vi "Get COM List.vi"(8 "error in (no error)":errorcluster) -> (0 "error out":errorcluster, 1 "raw string list":string, 2 "COM ports count":i32, 3 "COM list":T1[](array[typedef]))   [LabVIEW 2020, in "Get COM Descriptor.lvlib"]
doc: "Get list of available COM ports and their descriptors."
uses:
  Get COM Descriptor.lvlib
  COM port.ctl
  get_com_descriptor.dll
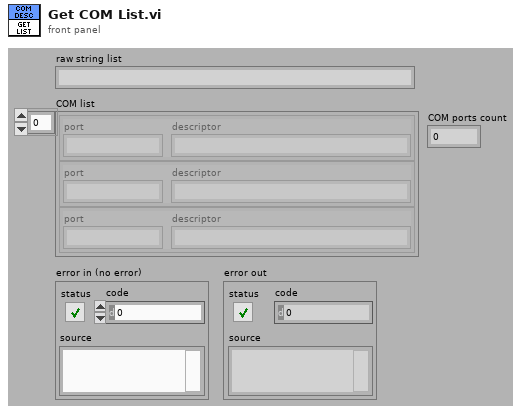
[diagram p1: front panel]
types:
  T1 = typedef "Get COM Descriptor.lvlib/COM port.ctl" = cluster{"port":string, "descriptor":string}
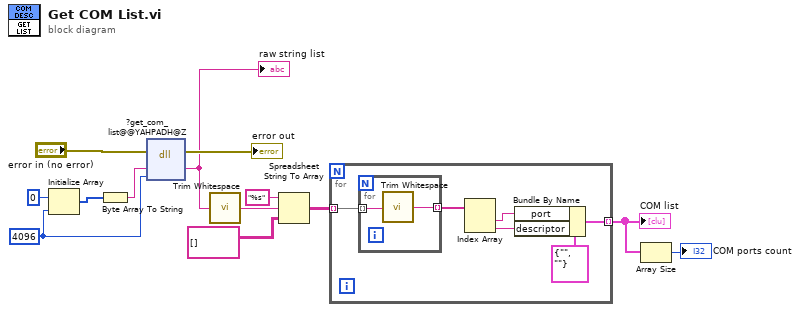
[diagram p0: block diagram]
diagram:
  w8 = 4096 ("dimension size")
  n1 = Initialize Array(u8 0 ("element"), w8) -> (w11:u8[])
  n2 = Byte Array To String(unsigned byte array=w11) -> (string=w9:string)
  n3 = dll-call lib="F:/z-bridge-v4/other/get_com_descriptor/get_com_descriptor.dll" fn="?get_com_list@@YAHPADH@Z"(error in="error in (no error)", "buf"=w9, "size"=w8) -> (error out=→"error out":errorcluster, "buf"=w7:string)  [unwired: 4 in, 1 out]
  "raw string list" <- w7
  n4 = call <vilib>:"Trim Whitespace.vi"("string"=w7) -> ("trimmed string"=w6:string)  [unwired: 1 in]
  n5 = Spreadsheet String To Array(format string="%s", spreadsheet string=w6, array type (2D Dbl)=string[][] []) -> (array=w3:string[][])  [unwired: 1 in]
  n6 = for {
    tunnel: w3 -> [w19] mode=indexing
    tunnel: [w14] -> w2 mode=indexing
    n7 = for {
      tunnel: w19 -> [w21] mode=indexing
      tunnel: [w20] -> w18 mode=indexing
      n8 = call <vilib>:"Trim Whitespace.vi"("string"=w21) -> ("trimmed string"=w20:string)  [unwired: 1 in]
    }
    n9 = Index Array(array=w18) -> (element #1=w16:string, element #2=w15:string)  [unwired: 2 in]
    n10 = Bundle By Name(cluster=T1 {"port"="", "descriptor"=""} ("COM port"), "port"=w16, "descriptor"=w15) -> (w14:T1)
  }
  "COM list" <- w2
  n11 = Array Size(array=w2) -> (size(s)=→"COM ports count":i32)
